vi "SPARC4_GEI.vi"() -> ()   [LabVIEW 2018]
uses:
  SPARC4_GUI/SPARC4_GUI.lvclass
  SPARC4_GUI/SPARC4_GUI.lvclass/SPARC4_GUI.ctl
  Channel GUI/Channel GUI.lvclass/Channel GUI.ctl
  Stream/Stream.lvclass/Stream.ctl
  Interface/Interface.lvclass/Interface.ctl
  Channel GUI/Channel GUI.lvclass
  Stream/Stream.lvclass
  State Machine/State Machine.lvclass
  Interface/Interface.lvclass
panel:
  out "Error":string
  in  "Tab Control 2":T1(tab)
  in  "#index":u16=1 step=1
  in  "Abort Acquisition":bool
  in  "Stop Acquisition":bool
  in  "# Sequences":u32=1 min=1
  in  "Cube Size  2":u16=1 min=1
  in  "SEND":bool
  out "Response:":string
  in  "Command:":string
  out "Current image":string="CH1"
  out "CCD Status":string
  out "Current TEXP":sgl
  out "Exposing":bool
  out "Temperature 2":i16
  out "Serial Number":u16
  out "Temperature Status":string
  in  "Exp Time 2":sgl=1e-05 min=1e-05
  out "Exposições realizadas":u16(slide) max=2 scale=0.0..1.0
  in  "Acquire":bool
  out "Initialization":bool
  in  "Stop Application":bool
  in  "Shutter Mode":u8(ring)=2 items=["Fully Auto", "OPEN", "CLOSED"]
  in  "Cube Size":u16=1 min=1
  in  "Cooler ON/OFF":u16(ring) items=["Cooler OFF", "Cooler ON"]
  in  "Temperature":i16=20 min=-80 max=20
  in  "Exposure Time":sgl=1e-05 min=1e-05
  in  "Readout Rate":u8(ring) items=["30 MHz", "20 MHz", "10 MHz", "  1 MHz"]
  in  "Pre-amp gain":u8(ring) items=["Gain 1", "Gain 2"]
  in  "EM Gain":u16=2
  in  "EM Mode":u8(ring) items=["Electron Multiplying", "Conventional"]
  in  "Sub Image":T2(radio)=enum."1024 x 1024"
  in  "Final Line":u16=1024
  in  "Final Column":u16=1024
  in  "Initial Cloumn":u16=1
  in  "Initial Line":u16=1
  in  "Binning":u16=1
  in  "Observation Setup":T3={"Night Directory:"="C:\\Users\\observer\\Desktop\\Imagens\\", "Base Name:"="IMG", "IP Address:"="//localhost", "Observation Title"="Observation", "Comment"="Write your comment"}
  # "SPARC4 \nGraphical Engineering Interface (GEI)"
  # "Temperature & Shutter"
  # "Timings"
  # "Horizontal pixel shift"
  # "EM Mode"
  # "Sub Image & Binning"
  # "Observation Setup"
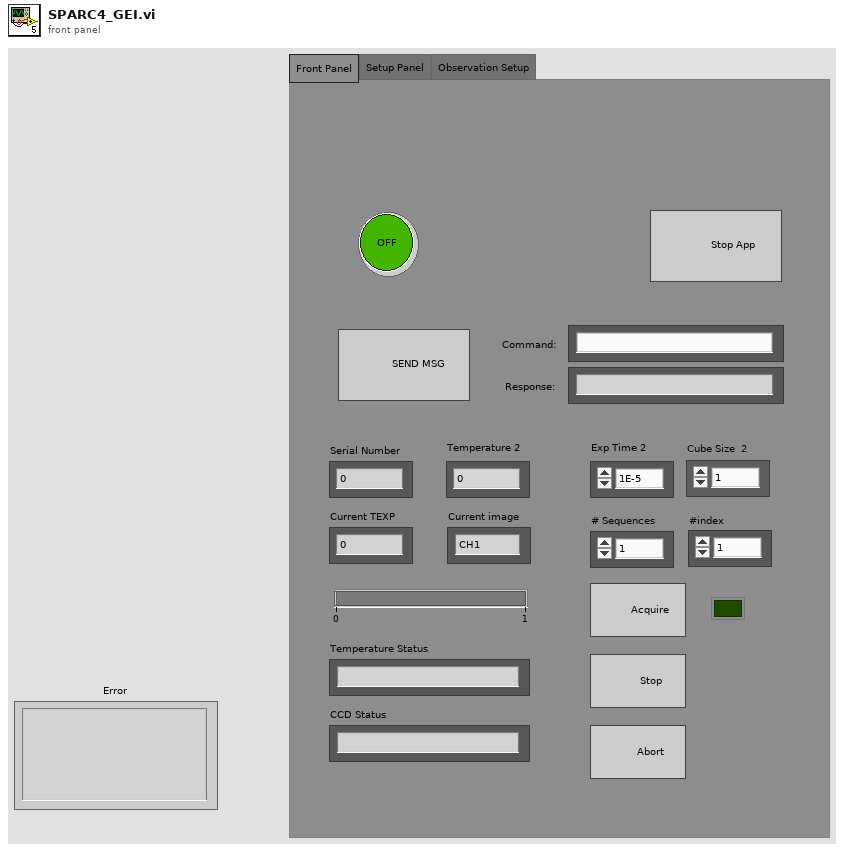
[diagram p1: front panel]
types:
  T1 = enum32{"Front Panel", "Setup Panel", "Observation Setup"}
  T2 = enum32{"256 x 256", "512 x 512", "1024 x 1024", "Custom"}
  T3 = cluster{"Night Directory:":string, "Base Name:":string, "IP Address:":string, "Observation Title":string, "Comment":string}
  T4 = cluster{"Exposure Time":sgl, "Pre-amp gain":u8, "Readout Rate":u8, "EM Mode":u8, "EM Gain":u16, "Binning":u16, "Initial Line":u16, "Initial Cloumn":u16, "Final Line":u16, "Final Column":u16, "Kinetic Series Length":u32, "Shutter Mode":u8, "Cooler ON/OFF":u16, "Temperature":i8, "Image Name":string, "Image Path":string, "#Images":u32, "#index":u16, "Trigger":u16}
  T5 = enum8{"Enabled", "Disabled", "Disabled and Grayed Out"}
  T6 = cluster{"Current Exptime":sgl, "Exposures Done":u16, "Last Image":string, "Disk Space":u16, "Exptime":sgl, "NImages":u16, "#index":u16, "File Base Name":string, "Image Path":string, "OBS Title":string, "Comment":string, "DS9":bool, "Cam_Status":string}
  T7 = cluster{"Initialization":bool, "Serial Number":u16}
  T8 = cluster{"Current Temperature":i16, "Temperatue Status":string}
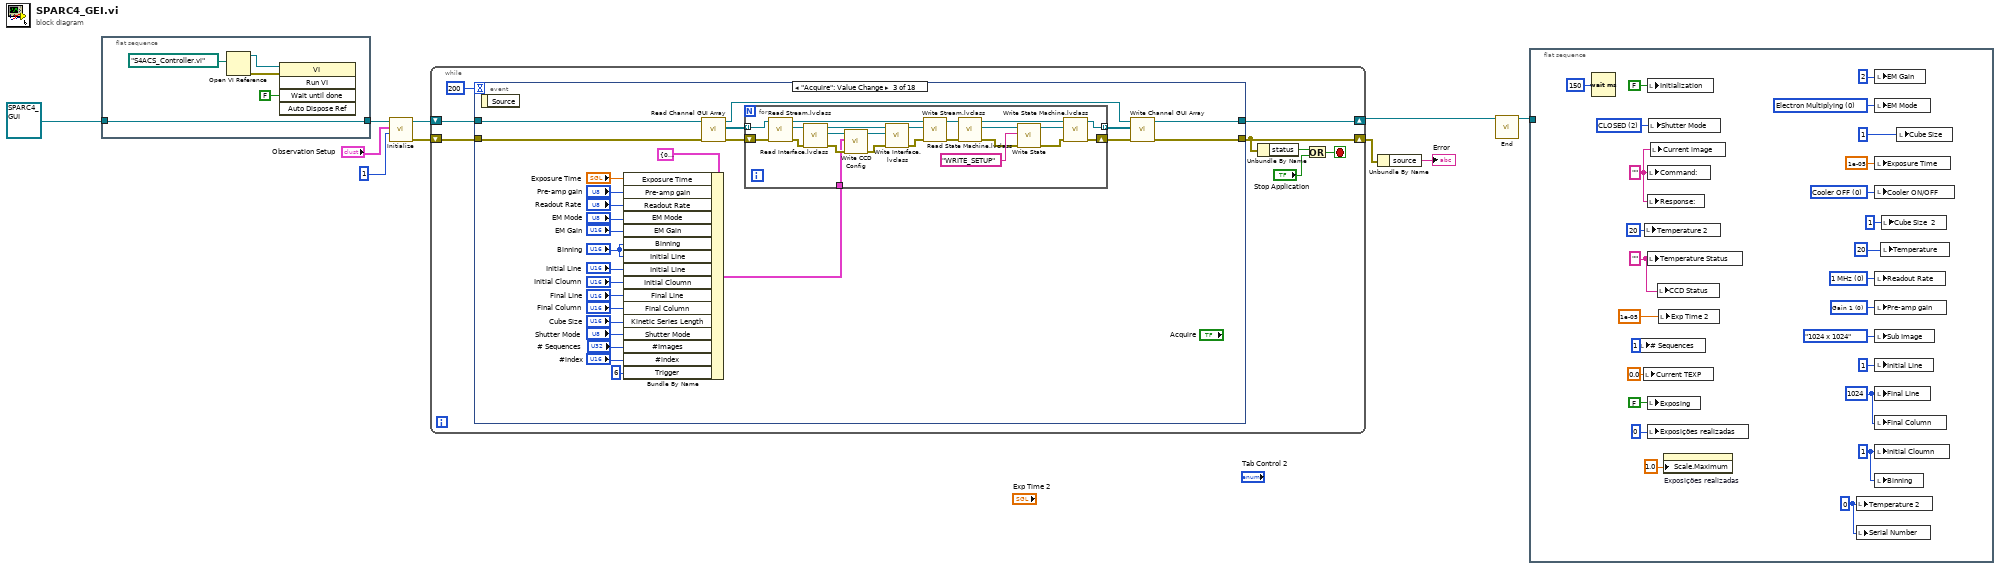
[diagram p0: block diagram]
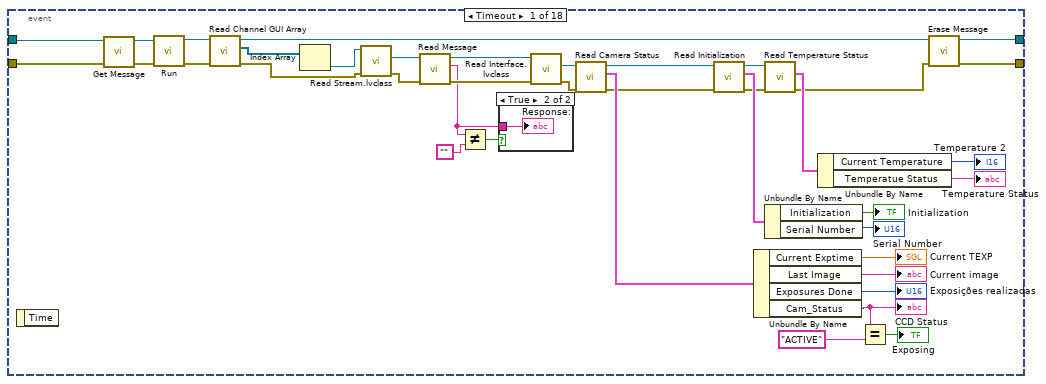
[diagram p2: hidden frame]
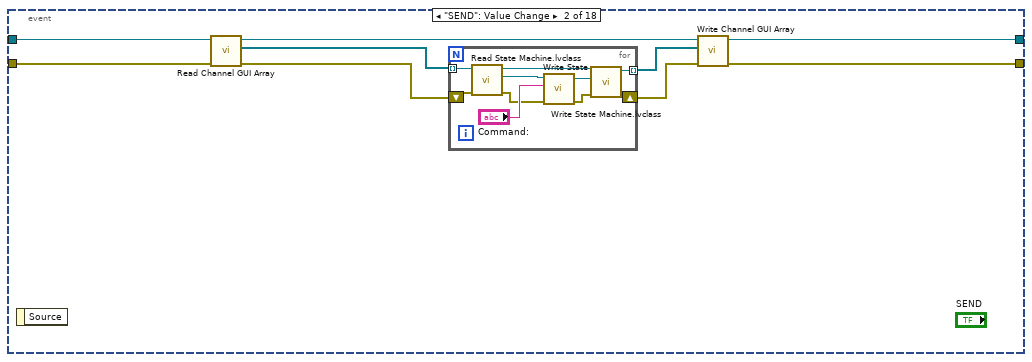
[diagram p4: hidden frame]
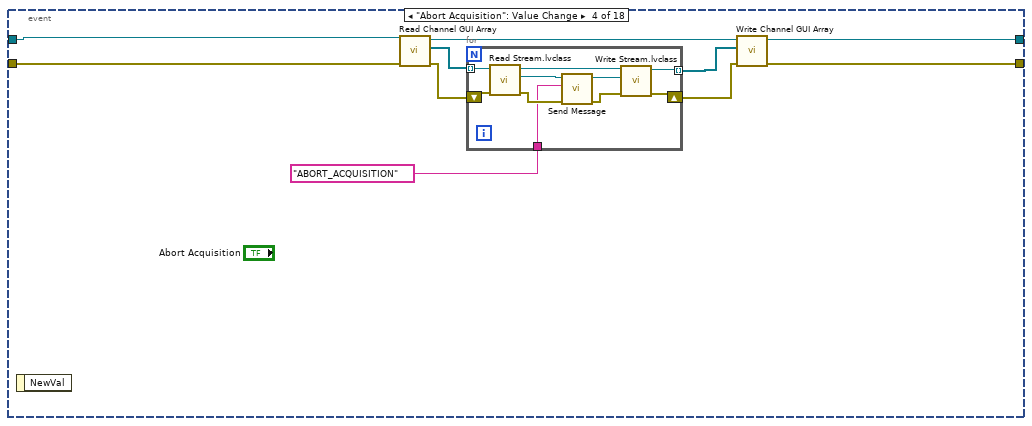
[diagram p5: hidden frame]
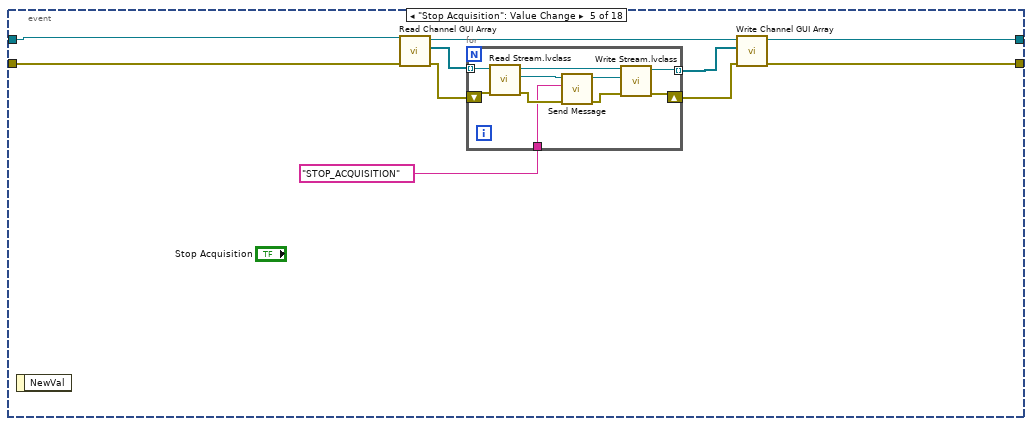
[diagram p6: hidden frame]
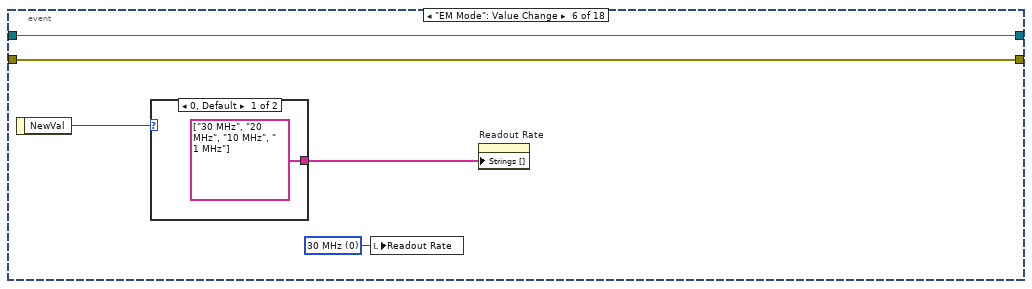
[diagram p7: hidden frame]
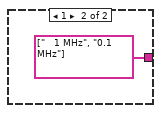
[diagram p8: hidden frame]
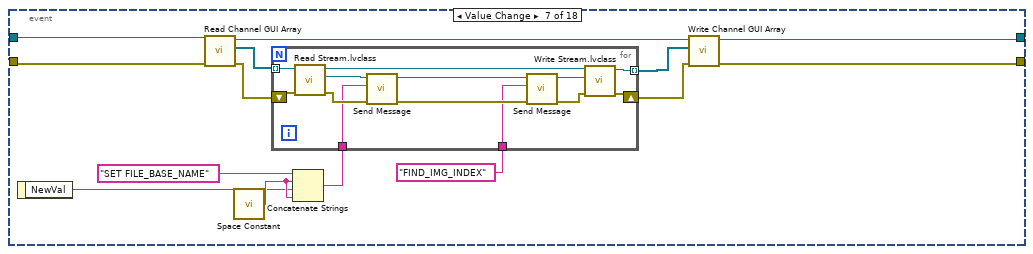
[diagram p9: hidden frame]
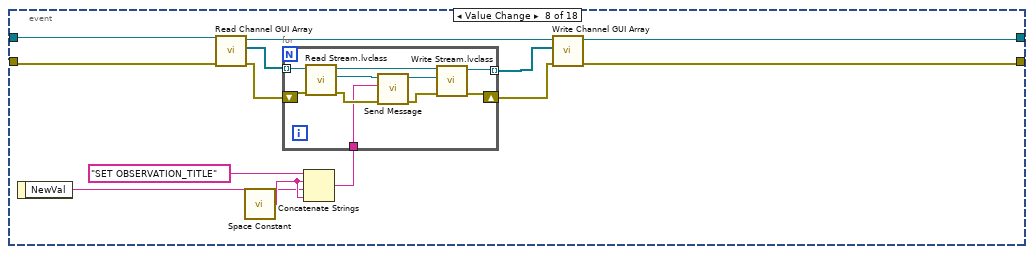
[diagram p10: hidden frame]
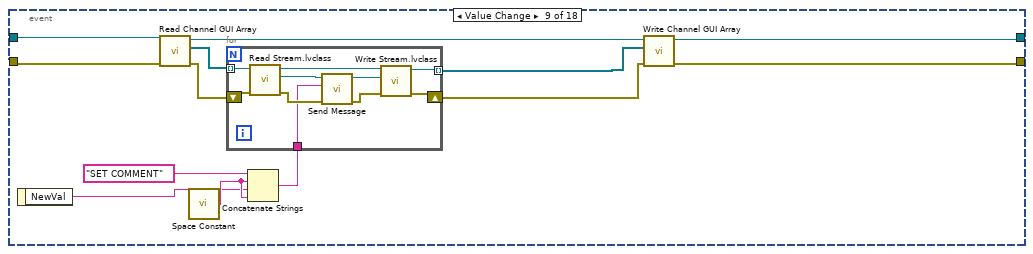
[diagram p11: hidden frame]
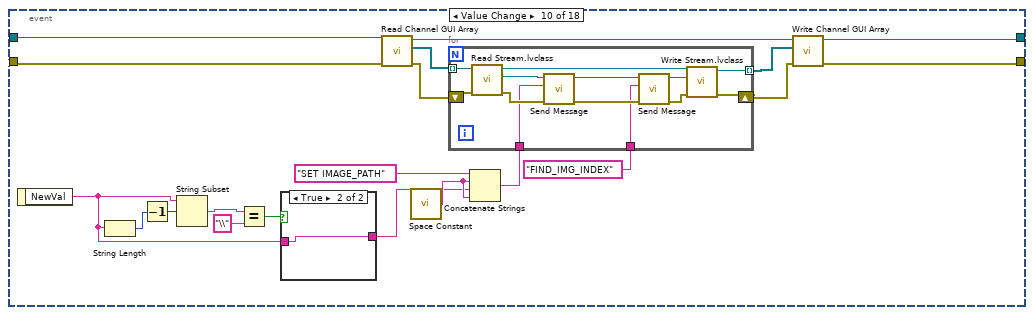
[diagram p12: hidden frame]
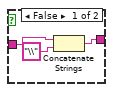
[diagram p13: hidden frame]
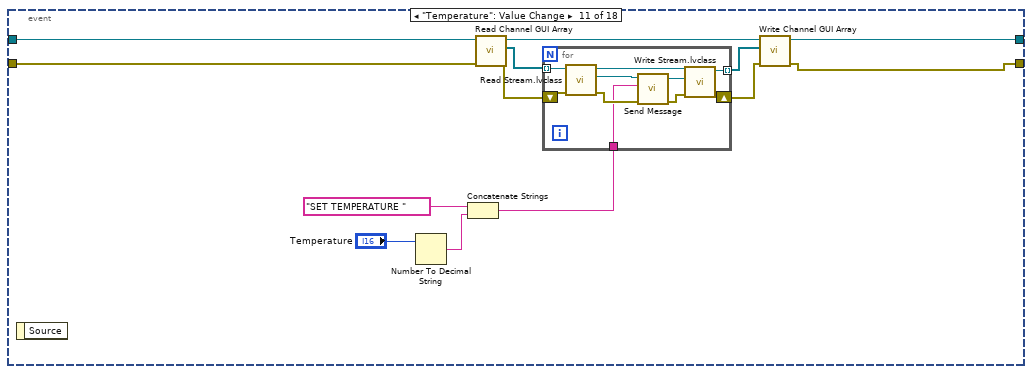
[diagram p14: hidden frame]
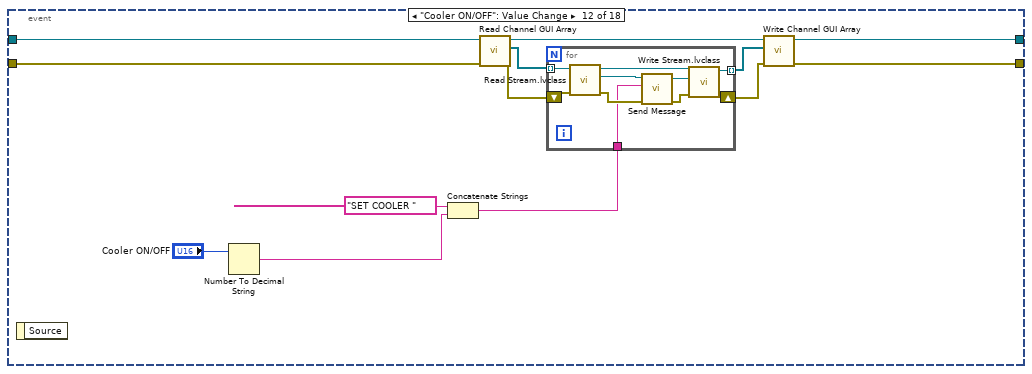
[diagram p15: hidden frame]
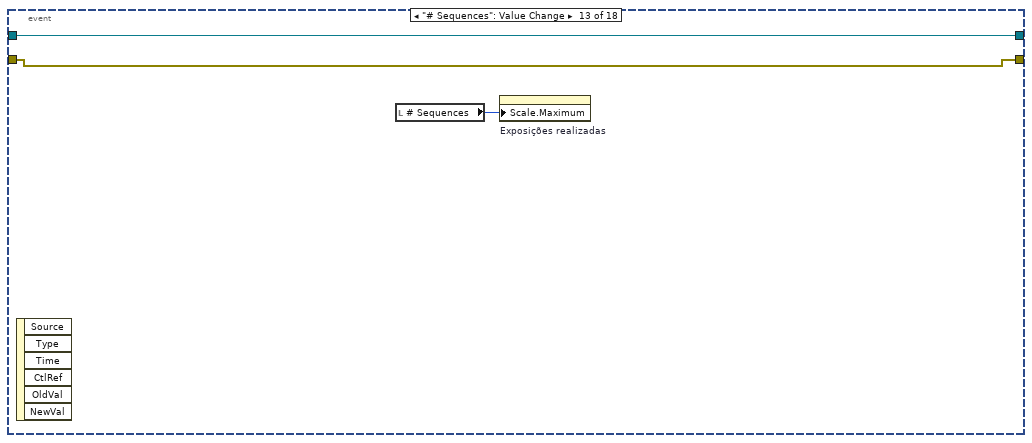
[diagram p16: hidden frame]
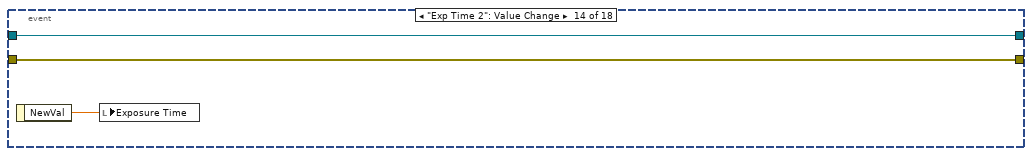
[diagram p17: hidden frame]
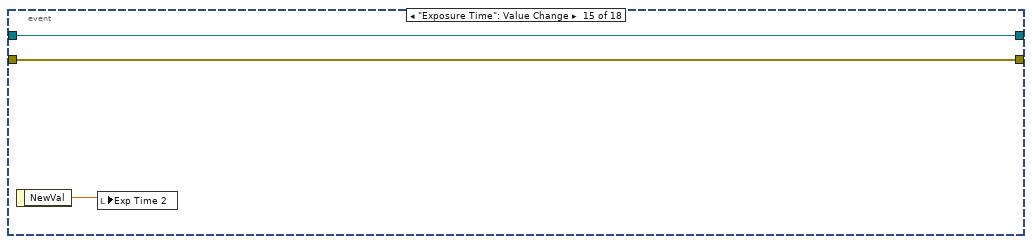
[diagram p18: hidden frame]
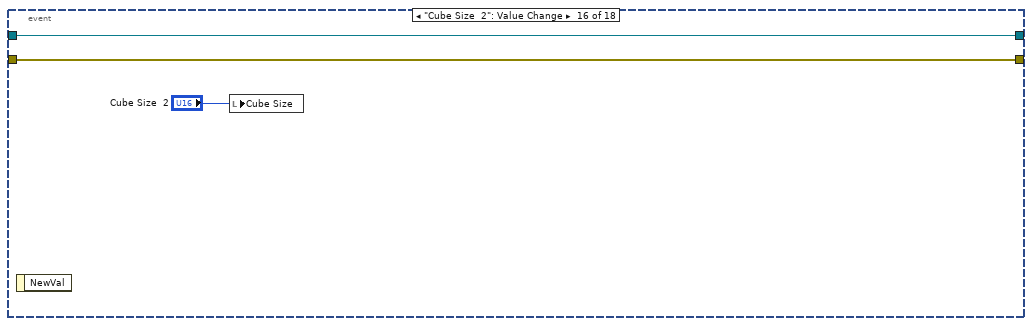
[diagram p19: hidden frame]
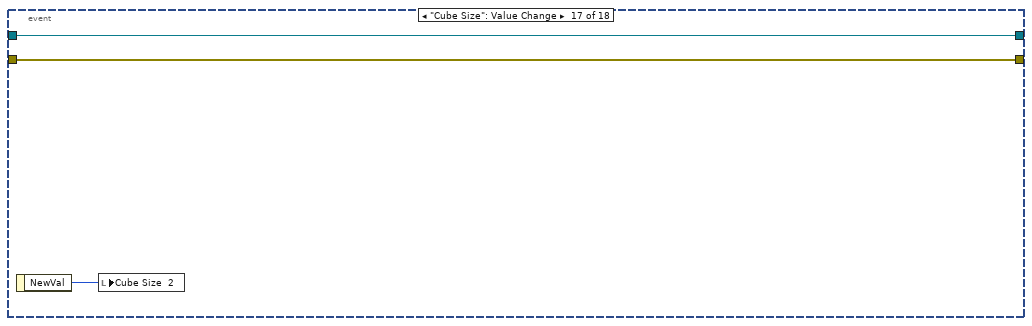
[diagram p20: hidden frame]
diagram:
  n1 = flat-sequence {
    tunnel: refnum<class "SPARC4_GUI.lvclass"> refnum ("SPARC4_GUI.lvclass") -> [w11]
    tunnel: [w11] -> w8
    frame #0 {
      n2 = Open VI Reference(vi path=path "S4ACS_Controller.vi") -> (vi reference=w15:refnum<vi>, error out=w14:errorcluster)  [unwired: 5 in]
      n3 = invoke class="VI" method="Run VI"(reference=w15, error in=w14, "Wait until done"=FALSE ("Wait Until Done")) -> ()  [unwired: 2 in, 5 out]
    }
  }
  n4 = call "Initialize.vi"("Camera ID"=1, "Observation Setup"="Observation Setup", "SPARC4_GUI in"=w8) -> ("error out"=w10:errorcluster, "SPARC4_GUI out"=w9:refnum<class "SPARC4_GUI.lvclass">)  [unwired: 7 in]
  n5 = while {
    shift-right: [w16] -> w4
    shift-left: w10 -> [w17]
    shift-right: [w19] -> w5
    shift-left: w9 -> [w18]
    stop <- w22 stop-if-true
    n6 = event shown="[2] \"Acquire\": Value Change" {
      selector: _ -> [_ _ _ _ _ _ _ _ _ _ _ _ _ _ _ _ _ _]
      dyn-events: _ -> [_ _ _ _ _ _ _ _ _ _ _ _ _ _ _ _ _ _]
      timeout: 200 -> [_ _ _ _ _ _ _ _ _ _ _ _ _ _ _ _ _ _]
      tunnel: w17 -> [w53 w71 w95 w135 w155 w175 w183 w209 w232 w256 w291 w315 w336 w339 w342 w345 w348 w366]
      tunnel: [w32 w64 w93 w133 w153 w175 w189 w215 w238 w262 w297 w313 w336 w339 w342 w345 w348 w364] -> w16
      tunnel: w18 -> [w54 w72 w96 w136 w156 w176 w182 w208 w231 w255 w290 w316 w337 w340 w341 w346 w349 w367]
      tunnel: [w33 w65 w94 w134 w154 w176 w190 w216 w239 w263 w298 w314 w337 w340 w341 w346 w349 w365] -> w19
      event Timeout {
        n7 = event-data() -> ()  [unwired: 1 in, 1 out]
        n8 = call "Get Message.vi"("error in (no error)"=w53, "SPARC4_GUI in"=w54) -> ("error out"=w56:errorcluster, "SPARC4_GUI out"=w55:refnum<class "SPARC4_GUI.lvclass">)  [unwired: 8 in]
        n9 = call "Run.vi"("error in (no error)"=w56, "SPARC4_GUI in"=w55) -> ("error out"=w61:errorcluster, "SPARC4_GUI out"=w60:refnum<class "SPARC4_GUI.lvclass">)  [unwired: 8 in]
        n10 = call "Read Channel GUI Array.vi"("error in (no error)"=w61, "SPARC4_GUI in"=w60) -> ("error out"=w35:errorcluster, "Channel GUI Array"=w37:refnum<class "Channel GUI.lvclass">[], "SPARC4_GUI out"=w31:refnum<class "SPARC4_GUI.lvclass">)  [unwired: 7 in]
        n11 = Index Array(array=w37) -> (element=w36:refnum<class "Channel GUI.lvclass">)  [unwired: 1 in]
        n12 = call "Read Stream.lvclass.vi"("error in (no error)"=w35, "Channel GUI in"=w36) -> ("error out"=w34:errorcluster, "Stream.lvclass"=w38:refnum<class "Stream.lvclass">)  [unwired: 7 in, 1 out]
        n13 = call "Read Message.vi"("error in (no error)"=w34, "Stream in"=w38) -> ("error out"=w41:errorcluster, "Message"=w28:string, "Stream out"=w42:refnum<class "Stream.lvclass">)  [unwired: 7 in]
        n14 = Not Equal?(x=w28, y="") -> (x != y?=w29:bool)
        n15 = case shown="True" w29 {
          tunnel: w28 -> [_ w63]
          frame False {
          }
          frame True {
            "Response:" <- w63
          }
        }
        n16 = call "Read Interface.lvclass.vi"("error in (no error)"=w41, "Stream in"=w42) -> ("error out"=w58:errorcluster, "Interface.lvclass"=w59:refnum<class "Interface.lvclass">)  [unwired: 7 in, 1 out]
        n17 = call "Read Camera Status.vi"("error in (no error)"=w58, "Interface in"=w59) -> ("error out"=w52:errorcluster, "Camera Status"=w57:T6, "Interface out"=w51:refnum<class "Interface.lvclass">)  [unwired: 7 in]
        n18 = call "Read Initialization.vi"("error in (no error)"=w52, "Interface in"=w51) -> ("error out"=w47:errorcluster, "Initialization"=w50:T7, "Interface out"=w46:refnum<class "Interface.lvclass">)  [unwired: 7 in]
        n19 = Unbundle By Name(w57) -> ("Current Exptime"=→"Current TEXP":sgl, "Last Image"=→"Current image":string, "Exposures Done"=→"Exposições realizadas":u16, "Cam_Status"=w26:string)
        "CCD Status" <- w26
        n20 = call "Read Temperature Status.vi"("error in (no error)"=w47, "Interface in"=w46) -> ("error out"=w30:errorcluster, "Temperature Status"=w45:T8)  [unwired: 7 in, 1 out]
        n21 = Unbundle By Name(w50) -> ("Initialization"=→"Initialization":bool, "Serial Number"=→"Serial Number":u16)
        n22 = Unbundle By Name(w45) -> ("Current Temperature"=→"Temperature 2":i16, "Temperatue Status"=→"Temperature Status":string)
        n23 = Equal?(x=w26, y="ACTIVE") -> (x = y?=→"Exposing":bool)
        n24 = call "Erase Message.vi"("error in (no error)"=w30, "SPARC4_GUI in"=w31) -> ("error out"=w32:errorcluster, "SPARC4_GUI out"=w33:refnum<class "SPARC4_GUI.lvclass">)  [unwired: 8 in]
      }
      event "SEND": Value Change {
        n25 = event-data() -> ()  [unwired: 1 in, 1 out]
        n26 = call "Read Channel GUI Array.vi"("error in (no error)"=w71, "SPARC4_GUI in"=w72) -> ("error out"=w67:errorcluster, "Channel GUI Array"=w70:refnum<class "Channel GUI.lvclass">[], "SPARC4_GUI out"=w66:refnum<class "SPARC4_GUI.lvclass">)  [unwired: 7 in]
        n27 = for {
          tunnel: w70 -> [w80] mode=indexing
          tunnel: [w81] -> w69 mode=indexing
          shift-right: [w75] -> w68
          shift-left: w67 -> [w74]
          n28 = call "Read State Machine.lvclass.vi"("error in (no error)"=w74, "Channel GUI in"=w80) -> ("error out"=w77:errorcluster, "State Machine.lvclass"=w78:refnum<class "State Machine.lvclass">, "Channel GUI out"=w79:refnum<class "Channel GUI.lvclass">)  [unwired: 7 in]
          n29 = call-dynamic "Write State.vi"("error in (no error)"=w77, "State"="Command:", "State Machine in"=w78) -> ("error out"=w76:errorcluster, "State Machine out"=w73:refnum<class "State Machine.lvclass">)  [unwired: 7 in]
          n30 = call "Write State Machine.lvclass.vi"("error in (no error)"=w76, "State Machine.lvclass"=w73, "Channel GUI in"=w79) -> ("error out"=w75:errorcluster, "Channel GUI out"=w81:refnum<class "Channel GUI.lvclass">)  [unwired: 7 in]
        }
        n31 = call "Write Channel GUI Array.vi"("error in (no error)"=w68, "Channel GUI Array"=w69, "SPARC4_GUI in"=w66) -> ("error out"=w64:errorcluster, "SPARC4_GUI out"=w65:refnum<class "SPARC4_GUI.lvclass">)  [unwired: 7 in]
      }
      event "Acquire": Value Change {
        n32 = event-data() -> ()  [unwired: 1 in, 1 out]
        n33 = Bundle By Name(cluster=T4 {"Exposure Time"=0.0, "Pre-amp gain"=0, "Readout Rate"=0, "EM Mode"=0, "EM Gain"=0, "Binning"=0, "Initial Line"=0, "Initial Cloumn"=0, "Final Line"=0, "Final Column"=0, "Kinetic Series Length"=0, "Shutter Mode"=0, "Cooler ON/OFF"=0, "Temperature"=0, "Image Name"="", "Image Path"="", "#Images"=0, "#index"=0, "Trigger"=0} ("CCD Config"), "Exposure Time"="Exposure Time", "Pre-amp gain"="Pre-amp gain", "Readout Rate"="Readout Rate", "EM Mode"="EM Mode", "EM Gain"="EM Gain", "Binning"="Binning", "Initial Line"="Binning", "Initial Line"="Initial Line", "Initial Cloumn"="Initial Cloumn", "Final Line"="Final Line", "Final Column"="Final Column", "Kinetic Series Length"="Cube Size", "Shutter Mode"="Shutter Mode", "#Images"="# Sequences", "#index"="#index", "Trigger"=u16 6) -> (w108:T4)
        n34 = call "Read Channel GUI Array.vi"("error in (no error)"=w95, "SPARC4_GUI in"=w96) -> ("error out"=w89:errorcluster, "Channel GUI Array"=w90:refnum<class "Channel GUI.lvclass">[], "SPARC4_GUI out"=w86:refnum<class "SPARC4_GUI.lvclass">)  [unwired: 7 in]
        n35 = for {
          tunnel: w108 -> [w129]
          tunnel: w90 -> [w112] mode=indexing
          tunnel: [w110] -> w88 mode=indexing
          shift-right: [w109] -> w87
          shift-left: w89 -> [w111]
          n36 = call "Read Stream.lvclass.vi"("error in (no error)"=w111, "Channel GUI in"=w112) -> ("error out"=w123:errorcluster, "Stream.lvclass"=w124:refnum<class "Stream.lvclass">, "Channel GUI out"=w120:refnum<class "Channel GUI.lvclass">)  [unwired: 7 in]
          n37 = call "Read Interface.lvclass.vi"("error in (no error)"=w123, "Stream in"=w124) -> ("error out"=w130:errorcluster, "Interface.lvclass"=w131:refnum<class "Interface.lvclass">, "Stream out"=w128:refnum<class "Stream.lvclass">)  [unwired: 7 in]
          n38 = call "Write CCD Config.vi"("error in (no error)"=w130, "CCD Config"=w129, "Interface in"=w131) -> ("error out"=w126:errorcluster, "Interface out"=w125:refnum<class "Interface.lvclass">)  [unwired: 7 in]
          n39 = call "Write Interface.lvclass.vi"("error in (no error)"=w126, "Interface.lvclass"=w125, "Stream in"=w128) -> ("error out"=w122:errorcluster, "Stream out"=w121:refnum<class "Stream.lvclass">)  [unwired: 7 in]
          n40 = call "Write Stream.lvclass.vi"("error in (no error)"=w122, "Stream.lvclass"=w121, "Channel GUI in"=w120) -> ("error out"=w119:errorcluster, "Channel GUI out"=w118:refnum<class "Channel GUI.lvclass">)  [unwired: 7 in]
          n41 = call "Read State Machine.lvclass.vi"("error in (no error)"=w119, "Channel GUI in"=w118) -> ("error out"=w113:errorcluster, "State Machine.lvclass"=w116:refnum<class "State Machine.lvclass">, "Channel GUI out"=w117:refnum<class "Channel GUI.lvclass">)  [unwired: 7 in]
          n42 = call-dynamic "Write State.vi"("error in (no error)"=w113, "State"="WRITE_SETUP", "State Machine in"=w116) -> ("error out"=w114:errorcluster, "State Machine out"=w115:refnum<class "State Machine.lvclass">)  [unwired: 7 in]
          n43 = call "Write State Machine.lvclass.vi"("error in (no error)"=w114, "State Machine.lvclass"=w115, "Channel GUI in"=w117) -> ("error out"=w109:errorcluster, "Channel GUI out"=w110:refnum<class "Channel GUI.lvclass">)  [unwired: 7 in]
        }
        n44 = call "Write Channel GUI Array.vi"("error in (no error)"=w87, "Channel GUI Array"=w88, "SPARC4_GUI in"=w86) -> ("error out"=w93:errorcluster, "SPARC4_GUI out"=w94:refnum<class "SPARC4_GUI.lvclass">)  [unwired: 7 in]
      }
      event "Abort Acquisition": Value Change {
        n45 = event-data() -> ()  [unwired: 1 in, 1 out]
        n46 = call "Read Channel GUI Array.vi"("error in (no error)"=w135, "SPARC4_GUI in"=w136) -> ("error out"=w137:errorcluster, "Channel GUI Array"=w140:refnum<class "Channel GUI.lvclass">[], "SPARC4_GUI out"=w141:refnum<class "SPARC4_GUI.lvclass">)  [unwired: 7 in]
        n47 = for {
          tunnel: w140 -> [w150] mode=indexing
          tunnel: [w151] -> w139 mode=indexing
          shift-right: [w146] -> w138
          shift-left: w137 -> [w145]
          tunnel: "ABORT_ACQUISITION" ("Message") -> [w144]
          n48 = call "Read Stream.lvclass.vi"("error in (no error)"=w145, "Channel GUI in"=w150) -> ("error out"=w147:errorcluster, "Stream.lvclass"=w148:refnum<class "Stream.lvclass">, "Channel GUI out"=w149:refnum<class "Channel GUI.lvclass">)  [unwired: 7 in]
          n49 = call "Send Message.vi"("error in (no error)"=w147, "Message"=w144, "Stream in"=w148) -> ("error out"=w143:errorcluster, "Stream out"=w142:refnum<class "Stream.lvclass">)  [unwired: 7 in]
          n50 = call "Write Stream.lvclass.vi"("error in (no error)"=w143, "Stream.lvclass"=w142, "Channel GUI in"=w149) -> ("error out"=w146:errorcluster, "Channel GUI out"=w151:refnum<class "Channel GUI.lvclass">)  [unwired: 7 in]
        }
        n51 = call "Write Channel GUI Array.vi"("error in (no error)"=w138, "Channel GUI Array"=w139, "SPARC4_GUI in"=w141) -> ("error out"=w133:errorcluster, "SPARC4_GUI out"=w134:refnum<class "SPARC4_GUI.lvclass">)  [unwired: 7 in]
      }
      event "Stop Acquisition": Value Change {
        n52 = event-data() -> ()  [unwired: 1 in, 1 out]
        n53 = call "Read Channel GUI Array.vi"("error in (no error)"=w155, "SPARC4_GUI in"=w156) -> ("error out"=w157:errorcluster, "Channel GUI Array"=w160:refnum<class "Channel GUI.lvclass">[], "SPARC4_GUI out"=w161:refnum<class "SPARC4_GUI.lvclass">)  [unwired: 7 in]
        n54 = for {
          tunnel: w160 -> [w170] mode=indexing
          tunnel: [w171] -> w159 mode=indexing
          shift-right: [w166] -> w158
          shift-left: w157 -> [w165]
          tunnel: "STOP_ACQUISITION" ("Message") -> [w164]
          n55 = call "Read Stream.lvclass.vi"("error in (no error)"=w165, "Channel GUI in"=w170) -> ("error out"=w167:errorcluster, "Stream.lvclass"=w168:refnum<class "Stream.lvclass">, "Channel GUI out"=w169:refnum<class "Channel GUI.lvclass">)  [unwired: 7 in]
          n56 = call "Send Message.vi"("error in (no error)"=w167, "Message"=w164, "Stream in"=w168) -> ("error out"=w163:errorcluster, "Stream out"=w162:refnum<class "Stream.lvclass">)  [unwired: 7 in]
          n57 = call "Write Stream.lvclass.vi"("error in (no error)"=w163, "Stream.lvclass"=w162, "Channel GUI in"=w169) -> ("error out"=w166:errorcluster, "Channel GUI out"=w171:refnum<class "Channel GUI.lvclass">)  [unwired: 7 in]
        }
        n58 = call "Write Channel GUI Array.vi"("error in (no error)"=w158, "Channel GUI Array"=w159, "SPARC4_GUI in"=w161) -> ("error out"=w153:errorcluster, "SPARC4_GUI out"=w154:refnum<class "SPARC4_GUI.lvclass">)  [unwired: 7 in]
      }
      event "EM Mode": Value Change {
        w172 = u8 0 items=["30 MHz", "20 MHz", "10 MHz", "1 MHz"] ("Readout Rate")
        n59 = event-data() -> ("NewVal"=w173:u8)  [unwired: 1 in]
        n60 = case shown="0, Default" w173 {
          tunnel: [string[] ["30 MHz", "20 MHz", "10 MHz", "  1 MHz"] string[] ["   1 MHz", "0.1 MHz"]] -> w174
          frame 0, Default {
          }
          frame 1 {
          }
        }
        n61 = local write "Readout Rate"(w172) -> ()
        n62 = property on="Readout Rate" class="Ring (strict)"("Strings []"=w174) -> ()  [unwired: 2 in, 2 out]
      }
      event "Observation Setup.Base Name:": Value Change {
        n63 = event-data() -> ("NewVal"=w179:string)  [unwired: 1 in]
        n64 = call "Read Channel GUI Array.vi"("error in (no error)"=w183, "SPARC4_GUI in"=w182) -> ("error out"=w184:errorcluster, "Channel GUI Array"=w187:refnum<class "Channel GUI.lvclass">[], "SPARC4_GUI out"=w188:refnum<class "SPARC4_GUI.lvclass">)  [unwired: 7 in]
        n65 = call <vilib>:"Space Constant.vi"() -> ("String"=w191:string)
        n66 = Concatenate Strings("SET FILE_BASE_NAME" ("Message"), w191, w179, w191) -> (w181:string)
        n67 = for {
          tunnel: w187 -> [w204] mode=indexing
          tunnel: [w205] -> w186 mode=indexing
          shift-right: [w200] -> w185
          shift-left: w184 -> [w199]
          tunnel: w181 -> [w198]
          tunnel: "FIND_IMG_INDEX" ("Message") -> [w193]
          n68 = call "Read Stream.lvclass.vi"("error in (no error)"=w199, "Channel GUI in"=w204) -> ("error out"=w201:errorcluster, "Stream.lvclass"=w202:refnum<class "Stream.lvclass">, "Channel GUI out"=w203:refnum<class "Channel GUI.lvclass">)  [unwired: 7 in]
          n69 = call "Send Message.vi"("error in (no error)"=w201, "Message"=w198, "Stream in"=w202) -> ("error out"=w195:errorcluster, "Stream out"=w194:refnum<class "Stream.lvclass">)  [unwired: 7 in]
          n70 = call "Send Message.vi"("error in (no error)"=w195, "Message"=w193, "Stream in"=w194) -> ("error out"=w196:errorcluster, "Stream out"=w197:refnum<class "Stream.lvclass">)  [unwired: 7 in]
          n71 = call "Write Stream.lvclass.vi"("error in (no error)"=w196, "Stream.lvclass"=w197, "Channel GUI in"=w203) -> ("error out"=w200:errorcluster, "Channel GUI out"=w205:refnum<class "Channel GUI.lvclass">)  [unwired: 7 in]
        }
        n72 = call "Write Channel GUI Array.vi"("error in (no error)"=w185, "Channel GUI Array"=w186, "SPARC4_GUI in"=w188) -> ("error out"=w189:errorcluster, "SPARC4_GUI out"=w190:refnum<class "SPARC4_GUI.lvclass">)  [unwired: 7 in]
      }
      event "Observation Setup.Observation Title": Value Change {
        n73 = event-data() -> ("NewVal"=w206:string)  [unwired: 1 in]
        n74 = call "Read Channel GUI Array.vi"("error in (no error)"=w209, "SPARC4_GUI in"=w208) -> ("error out"=w210:errorcluster, "Channel GUI Array"=w213:refnum<class "Channel GUI.lvclass">[], "SPARC4_GUI out"=w214:refnum<class "SPARC4_GUI.lvclass">)  [unwired: 7 in]
        n75 = call <vilib>:"Space Constant.vi"() -> ("String"=w217:string)
        n76 = Concatenate Strings("SET OBSERVATION_TITLE" ("Message"), w217, w206, w217) -> (w207:string)
        n77 = for {
          tunnel: w213 -> [w227] mode=indexing
          tunnel: [w228] -> w212 mode=indexing
          shift-right: [w223] -> w211
          shift-left: w210 -> [w222]
          tunnel: w207 -> [w221]
          n78 = call "Read Stream.lvclass.vi"("error in (no error)"=w222, "Channel GUI in"=w227) -> ("error out"=w224:errorcluster, "Stream.lvclass"=w225:refnum<class "Stream.lvclass">, "Channel GUI out"=w226:refnum<class "Channel GUI.lvclass">)  [unwired: 7 in]
          n79 = call "Send Message.vi"("error in (no error)"=w224, "Message"=w221, "Stream in"=w225) -> ("error out"=w220:errorcluster, "Stream out"=w219:refnum<class "Stream.lvclass">)  [unwired: 7 in]
          n80 = call "Write Stream.lvclass.vi"("error in (no error)"=w220, "Stream.lvclass"=w219, "Channel GUI in"=w226) -> ("error out"=w223:errorcluster, "Channel GUI out"=w228:refnum<class "Channel GUI.lvclass">)  [unwired: 7 in]
        }
        n81 = call "Write Channel GUI Array.vi"("error in (no error)"=w211, "Channel GUI Array"=w212, "SPARC4_GUI in"=w214) -> ("error out"=w215:errorcluster, "SPARC4_GUI out"=w216:refnum<class "SPARC4_GUI.lvclass">)  [unwired: 7 in]
      }
      event "Observation Setup.Comment": Value Change {
        n82 = event-data() -> ("NewVal"=w229:string)  [unwired: 1 in]
        n83 = call "Read Channel GUI Array.vi"("error in (no error)"=w232, "SPARC4_GUI in"=w231) -> ("error out"=w233:errorcluster, "Channel GUI Array"=w236:refnum<class "Channel GUI.lvclass">[], "SPARC4_GUI out"=w237:refnum<class "SPARC4_GUI.lvclass">)  [unwired: 7 in]
        n84 = call <vilib>:"Space Constant.vi"() -> ("String"=w240:string)
        n85 = Concatenate Strings("SET COMMENT" ("Message"), w240, w229, w240) -> (w230:string)
        n86 = for {
          tunnel: w236 -> [w250] mode=indexing
          tunnel: [w251] -> w235 mode=indexing
          shift-right: [w246] -> w234
          shift-left: w233 -> [w245]
          tunnel: w230 -> [w244]
          n87 = call "Read Stream.lvclass.vi"("error in (no error)"=w245, "Channel GUI in"=w250) -> ("error out"=w247:errorcluster, "Stream.lvclass"=w248:refnum<class "Stream.lvclass">, "Channel GUI out"=w249:refnum<class "Channel GUI.lvclass">)  [unwired: 7 in]
          n88 = call "Send Message.vi"("error in (no error)"=w247, "Message"=w244, "Stream in"=w248) -> ("error out"=w243:errorcluster, "Stream out"=w242:refnum<class "Stream.lvclass">)  [unwired: 7 in]
          n89 = call "Write Stream.lvclass.vi"("error in (no error)"=w243, "Stream.lvclass"=w242, "Channel GUI in"=w249) -> ("error out"=w246:errorcluster, "Channel GUI out"=w251:refnum<class "Channel GUI.lvclass">)  [unwired: 7 in]
        }
        n90 = call "Write Channel GUI Array.vi"("error in (no error)"=w234, "Channel GUI Array"=w235, "SPARC4_GUI in"=w237) -> ("error out"=w238:errorcluster, "SPARC4_GUI out"=w239:refnum<class "SPARC4_GUI.lvclass">)  [unwired: 7 in]
      }
      event "Observation Setup.Night Directory:": Value Change {
        n91 = event-data() -> ("NewVal"=w253:string)  [unwired: 1 in]
        n92 = String Length(string=w253) -> (length=w266:i32)
        n93 = Decrement(x=w266) -> (x-1=w267:i32)
        n94 = String Subset(string=w253, offset (0)=w267) -> (substring=w268:string)  [unwired: 1 in]
        n95 = Equal?(x=w268, y="\\") -> (x = y?=w269:bool)
        n96 = case shown="True" w269 {
          tunnel: [w287 w288] -> w264
          tunnel: w253 -> [w285 w288]
          frame False {
            n97 = Concatenate Strings(w285, "\\") -> (w287:string)
          }
          frame True {
          }
        }
        n98 = call "Read Channel GUI Array.vi"("error in (no error)"=w256, "SPARC4_GUI in"=w255) -> ("error out"=w257:errorcluster, "Channel GUI Array"=w260:refnum<class "Channel GUI.lvclass">[], "SPARC4_GUI out"=w261:refnum<class "SPARC4_GUI.lvclass">)  [unwired: 7 in]
        n99 = call <vilib>:"Space Constant.vi"() -> ("String"=w270:string)
        n100 = Concatenate Strings("SET IMAGE_PATH" ("Message"), w270, w264, w270) -> (w254:string)
        n101 = for {
          tunnel: w260 -> [w283] mode=indexing
          tunnel: [w284] -> w259 mode=indexing
          shift-right: [w279] -> w258
          shift-left: w257 -> [w278]
          tunnel: w254 -> [w277]
          tunnel: "FIND_IMG_INDEX" ("Message") -> [w272]
          n102 = call "Read Stream.lvclass.vi"("error in (no error)"=w278, "Channel GUI in"=w283) -> ("error out"=w280:errorcluster, "Stream.lvclass"=w281:refnum<class "Stream.lvclass">, "Channel GUI out"=w282:refnum<class "Channel GUI.lvclass">)  [unwired: 7 in]
          n103 = call "Send Message.vi"("error in (no error)"=w280, "Message"=w277, "Stream in"=w281) -> ("error out"=w276:errorcluster, "Stream out"=w275:refnum<class "Stream.lvclass">)  [unwired: 7 in]
          n104 = call "Send Message.vi"("error in (no error)"=w276, "Message"=w272, "Stream in"=w275) -> ("error out"=w273:errorcluster, "Stream out"=w274:refnum<class "Stream.lvclass">)  [unwired: 7 in]
          n105 = call "Write Stream.lvclass.vi"("error in (no error)"=w273, "Stream.lvclass"=w274, "Channel GUI in"=w282) -> ("error out"=w279:errorcluster, "Channel GUI out"=w284:refnum<class "Channel GUI.lvclass">)  [unwired: 7 in]
        }
        n106 = call "Write Channel GUI Array.vi"("error in (no error)"=w258, "Channel GUI Array"=w259, "SPARC4_GUI in"=w261) -> ("error out"=w262:errorcluster, "SPARC4_GUI out"=w263:refnum<class "SPARC4_GUI.lvclass">)  [unwired: 7 in]
      }
      event "Temperature": Value Change {
        n107 = event-data() -> ()  [unwired: 1 in, 1 out]
        n108 = Number To Decimal String(number="Temperature") -> (decimal integer string=w300:string)  [unwired: 1 in]
        n109 = Concatenate Strings("SET TEMPERATURE " ("Message"), w300) -> (w289:string)
        n110 = call "Read Channel GUI Array.vi"("error in (no error)"=w291, "SPARC4_GUI in"=w290) -> ("error out"=w292:errorcluster, "Channel GUI Array"=w293:refnum<class "Channel GUI.lvclass">[], "SPARC4_GUI out"=w294:refnum<class "SPARC4_GUI.lvclass">)  [unwired: 7 in]
        n111 = for {
          tunnel: w293 -> [w310] mode=indexing
          tunnel: [w311] -> w295 mode=indexing
          shift-right: [w305] -> w296
          shift-left: w292 -> [w304]
          tunnel: w289 -> [w302]
          n112 = call "Read Stream.lvclass.vi"("error in (no error)"=w304, "Channel GUI in"=w310) -> ("error out"=w307:errorcluster, "Stream.lvclass"=w308:refnum<class "Stream.lvclass">, "Channel GUI out"=w309:refnum<class "Channel GUI.lvclass">)  [unwired: 7 in]
          n113 = call "Send Message.vi"("error in (no error)"=w307, "Message"=w302, "Stream in"=w308) -> ("error out"=w306:errorcluster, "Stream out"=w303:refnum<class "Stream.lvclass">)  [unwired: 7 in]
          n114 = call "Write Stream.lvclass.vi"("error in (no error)"=w306, "Stream.lvclass"=w303, "Channel GUI in"=w309) -> ("error out"=w305:errorcluster, "Channel GUI out"=w311:refnum<class "Channel GUI.lvclass">)  [unwired: 7 in]
        }
        n115 = call "Write Channel GUI Array.vi"("error in (no error)"=w296, "Channel GUI Array"=w295, "SPARC4_GUI in"=w294) -> ("error out"=w297:errorcluster, "SPARC4_GUI out"=w298:refnum<class "SPARC4_GUI.lvclass">)  [unwired: 7 in]
      }
      event "Cooler ON/OFF": Value Change {
        n116 = event-data() -> ()  [unwired: 1 in, 1 out]
        n117 = Number To Decimal String(number="Cooler ON/OFF") -> (decimal integer string=w322:string)  [unwired: 1 in]
        n118 = Concatenate Strings("SET COOLER ", w322) -> (w312:string)
        n119 = call "Read Channel GUI Array.vi"("error in (no error)"=w315, "SPARC4_GUI in"=w316) -> ("error out"=w317:errorcluster, "Channel GUI Array"=w318:refnum<class "Channel GUI.lvclass">[], "SPARC4_GUI out"=w319:refnum<class "SPARC4_GUI.lvclass">)  [unwired: 7 in]
        n120 = for {
          tunnel: w318 -> [w333] mode=indexing
          tunnel: [w334] -> w320 mode=indexing
          shift-right: [w328] -> w321
          shift-left: w317 -> [w327]
          tunnel: w312 -> [w325]
          n121 = call "Read Stream.lvclass.vi"("error in (no error)"=w327, "Channel GUI in"=w333) -> ("error out"=w330:errorcluster, "Stream.lvclass"=w331:refnum<class "Stream.lvclass">, "Channel GUI out"=w332:refnum<class "Channel GUI.lvclass">)  [unwired: 7 in]
          n122 = call "Send Message.vi"("error in (no error)"=w330, "Message"=w325, "Stream in"=w331) -> ("error out"=w329:errorcluster, "Stream out"=w326:refnum<class "Stream.lvclass">)  [unwired: 7 in]
          n123 = call "Write Stream.lvclass.vi"("error in (no error)"=w329, "Stream.lvclass"=w326, "Channel GUI in"=w332) -> ("error out"=w328:errorcluster, "Channel GUI out"=w334:refnum<class "Channel GUI.lvclass">)  [unwired: 7 in]
        }
        n124 = call "Write Channel GUI Array.vi"("error in (no error)"=w321, "Channel GUI Array"=w320, "SPARC4_GUI in"=w319) -> ("error out"=w313:errorcluster, "SPARC4_GUI out"=w314:refnum<class "SPARC4_GUI.lvclass">)  [unwired: 7 in]
      }
      event "# Sequences": Value Change {
        n125 = event-data() -> ()  [unwired: 1 in, 6 out]
        n126 = local read "# Sequences"() -> (w335:u32)
        n127 = property on="Exposições realizadas" class="Slide (strict)"("Scale.Maximum"=w335) -> ()  [unwired: 2 in, 2 out]
      }
      event "Exp Time 2": Value Change {
        n128 = event-data() -> ("NewVal"=w338:sgl)  [unwired: 1 in]
        n129 = local write "Exposure Time"(w338) -> ()
      }
      event "Exposure Time": Value Change {
        n130 = event-data() -> ("NewVal"=w343:sgl)  [unwired: 1 in]
        n131 = local write "Exp Time 2"(w343) -> ()
      }
      event "Cube Size  2": Value Change {
        n132 = event-data() -> ()  [unwired: 1 in, 1 out]
        n133 = local write "Cube Size"("Cube Size  2") -> ()
      }
      event "Cube Size": Value Change {
        n134 = event-data() -> ("NewVal"=w347:u16)  [unwired: 1 in]
        n135 = local write "Cube Size  2"(w347) -> ()
      }
      event "Sub Image": Value Change {
        w354 = 1024
        n136 = event-data() -> ()  [unwired: 1 in, 1 out]
        n137 = case shown="\"256 x 256\"" "Sub Image" {
          tunnel: [128 256 512 512] -> w358
          frame "256 x 256" {
          }
          frame "512 x 512" {
          }
          frame "1024 x 1024", Default {
          }
          frame "Custom" {
          }
        }
        n138 = case shown="\"1024 x 1024\", Default" "Sub Image" {
          tunnel: [T5."Disabled and Grayed Out" ("Disabled") T5."Enabled" ("Disabled")] -> w361
          frame "1024 x 1024", Default {
          }
          frame "Custom" {
          }
        }
        n139 = Divide(x=w354, y=2) -> (x/y=w357:dbl)
        n140 = Divide(x=w354, y=2) -> (x/y=w356:dbl)
        n141 = Add(x=w357, y=w358) -> (x+y=w350:dbl)
        n142 = Subtract(x=w357, y=w358) -> (x-y=w359:dbl)
        n143 = Subtract(x=w356, y=w358) -> (x-y=w360:dbl)
        n144 = Add(x=w356, y=w358) -> (x+y=w363:dbl)
        n145 = Increment(x=w359) -> (x+1=w362:dbl)
        n146 = Increment(x=w360) -> (x+1=w351:dbl)
        n147 = local write "Initial Cloumn"(w362) -> ()
        n148 = local write "Final Column"(w363) -> ()
        n149 = local write "Initial Line"(w351) -> ()
        n150 = local write "Final Line"(w350) -> ()
        n151 = property on="Initial Line" class="DigNum (strict)"("DisabledEnum"=w361) -> ()  [unwired: 2 in, 2 out]
        n152 = property on="Initial Cloumn" class="DigNum (strict)"("DisabledEnum"=w361) -> ()  [unwired: 2 in, 2 out]
        n153 = property on="Final Line" class="DigNum (strict)"("DisabledEnum"=w361) -> ()  [unwired: 2 in, 2 out]
        n154 = property on="Final Column" class="DigNum (strict)"("DisabledEnum"=w361) -> ()  [unwired: 2 in, 2 out]
        n155 = flat-sequence {
          tunnel: w366 -> [w384]
          tunnel: w367 -> [w385]
          tunnel: [w385] -> w365
          tunnel: [w384] -> w364
          frame #0 {
            w378 = cluster{dbl, dbl} {0.0, 0.0}
            n156 = local read "Initial Cloumn"() -> (w377:u16)
            n157 = local read "Final Column"() -> (w375:u16)
            n158 = local read "Final Line"() -> (w376:u16)
            n159 = local read "Final Line"() -> (w374:u16)
            n160 = Bundle(cluster=w378, w377, w376) -> (w383:cluster{dbl, dbl})
            n161 = Bundle(cluster=w378, w377, w374) -> (w382:cluster{dbl, dbl})
            n162 = Bundle(cluster=w378, w375, w374) -> (w381:cluster{dbl, dbl})
            n163 = Bundle(cluster=w378, w375, w376) -> (w380:cluster{dbl, dbl})
            n164 = Bundle(cluster=w378, w377, w376) -> (w379:cluster{dbl, dbl})
            n165 = Build Array(w383, w382, w381, w380, w379) -> ()  [unwired: 1 out]
          }
        }
      }
    }
    n166 = Unbundle By Name(w16) -> ("status"=w21:bool)
    n167 = Or(x=w21, y="Stop Application") -> (x .or. y?=w22:bool)
  }
  n168 = Unbundle By Name(w4) -> ("source"=→"Error":string)
  n169 = call "End.vi"("SPARC4_GUI in"=w5) -> ("SPARC4_GUI out"=w6:refnum<class "SPARC4_GUI.lvclass">)  [unwired: 9 in, 1 out]
  n170 = flat-sequence {
    tunnel: w6 -> [_]
    frame #0 {
      w388 = i16 0 ("Temperature 2")
      w392 = u8 2 items=["Fully Auto", "OPEN", "CLOSED"] ("Shutter Mode")
      w389 = "" ("Command:")
      w394 = u16 1024 ("Final Line")
      w393 = u16 1 ("Initial Cloumn")
      w397 = u8 0 items=["Gain 1", "Gain 2"] ("Pre-amp gain")
      w398 = u8 0 items=["1 MHz", "10 MHz", "20 MHz", "30 MHz"] ("Readout Rate")
      w400 = u16 0 items=["Cooler OFF", "Cooler ON"] ("Cooler ON/OFF")
      w403 = u8 0 items=["Electron Multiplying", "Conventional"] ("EM Mode")
      w390 = "" ("Temperature Status")
      n171 = Wait (ms)(milliseconds to wait=u32 150) -> ()  [unwired: 1 out]
      n172 = local write "# Sequences"(u32 1 ("# Ciclos")) -> ()
      n173 = local write "Current TEXP"(0.0 ("% Acquired")) -> ()
      n174 = local write "Temperature 2"(20 ("Temperature")) -> ()
      n175 = local write "Initialization"(FALSE ("Initialization")) -> ()
      n176 = local write "Command:"(w389) -> ()
      n177 = local write "Response:"(w389) -> ()
      n178 = local write "Temperature Status"(w390) -> ()
      n179 = local write "Exposing"(FALSE ("Exposing")) -> ()
      n180 = local write "Exposições realizadas"(u8 0 ("Exposições realizadas")) -> ()
      n181 = local write "Shutter Mode"(w392) -> ()
      n182 = local write "Current image"(w389) -> ()
      n183 = local write "CCD Status"(w390) -> ()
      n184 = local write "Exp Time 2"(1e-05 ("Exposure Time 2")) -> ()
      n185 = property on="Exposições realizadas" class="Slide (strict)"("Scale.Maximum"=1.0 ("Scale.Range:Maximum")) -> ()  [unwired: 2 in, 2 out]
      n186 = local write "Temperature 2"(w388) -> ()
      n187 = local write "Serial Number"(w388) -> ()
      n188 = local write "EM Gain"(u16 2 ("EM Gain")) -> ()
      n189 = local write "EM Mode"(w403) -> ()
      n190 = local write "Exposure Time"(1e-05 ("Exposure Time")) -> ()
      n191 = local write "Cooler ON/OFF"(w400) -> ()
      n192 = local write "Readout Rate"(w398) -> ()
      n193 = local write "Pre-amp gain"(w397) -> ()
      n194 = local write "Sub Image"(T2."1024 x 1024" ("Sub Image")) -> ()
      n195 = local write "Initial Line"(u16 1 ("Initial Line")) -> ()
      n196 = local write "Final Line"(w394) -> ()
      n197 = local write "Final Column"(w394) -> ()
      n198 = local write "Initial Cloumn"(w393) -> ()
      n199 = local write "Binning"(w393) -> ()
      n200 = local write "Temperature"(i16 20 ("Set temperature")) -> ()
      n201 = local write "Cube Size  2"(u16 1 ("Cube Size  2")) -> ()
      n202 = local write "Cube Size"(u16 1 ("Kinetic Series Length")) -> ()
    }
  }
